vi "Launch Actors.vi"() -> ()   [LabVIEW 2020]
uses:
  Form Server.lvclass
  C:/Program Files (x86)/National Instruments/LabVIEW 2020/vi.lib/ActorFramework/Actor/Actor.lvclass
  Form Configuration.lvclass
  ADODB.lvclass
  C:/Users/User/Desktop/Raman Program/Database OOP/source/Database/Database.lvclass
  Working Range.lvclass
  Panel Form Controller.lvclass
  TRExperimentsRaw.lvclass
  DataSets.lvclass
  Sample Chemical Formula.lvclass
  Samples.lvclass
  Solutions.lvclass
  Users.lvclass
  Form Configuration.lvclass/Form Configuration.ctl
  Open Form Msg.lvclass/Open Form Msg.ctl
  <vilib>/ActorFramework/Message Enqueuer/Message Enqueuer.lvclass/Message Enqueuer.ctl
  <vilib>/ActorFramework/Message Enqueuer/Enqueue.vi
  <vilib>/MGI/Panel Manager/Panel/Panel/Window/Window.lvclass
  C:/Program Files (x86)/National Instruments/LabVIEW 2020/vi.lib/MGI/Panel Manager/Panel/Panel/Panel.lvclass
  Open Form Msg.lvclass
  C:/Program Files (x86)/National Instruments/LabVIEW 2020/vi.lib/ActorFramework/Message/Message.lvclass
  <vilib>/ActorFramework/Stop Msg/Stop Msg.lvclass
  <vilib>/MGI/Panel Manager/Panel/Panel/Window/Window.vi
  <vilib>/ActorFramework/Message Priority Queue/Priority Enqueue.vi
  <vilib>/ActorFramework/Actor/Actor.lvclass
  <vilib>/MGI/Panel Manager/Panel/Panel.lvlib
panel:
  in  "stop":bool
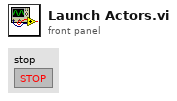
[diagram p1: front panel]
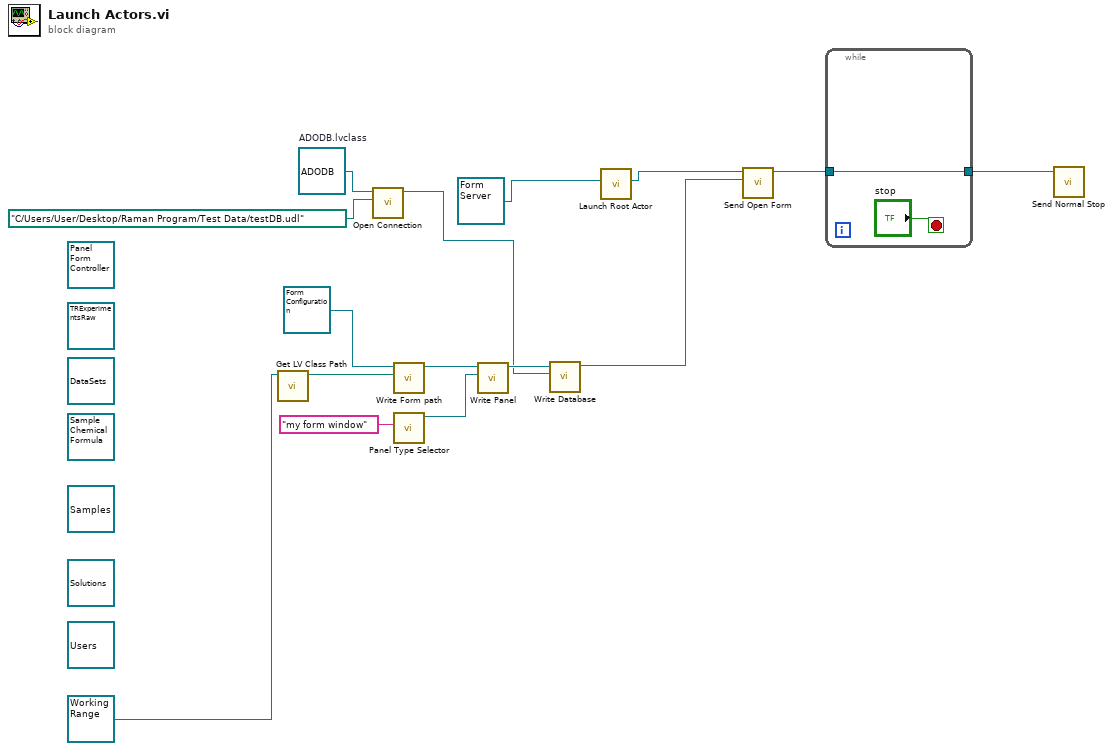
[diagram p0: block diagram]
diagram:
  (unwired) refnum<class "Users.lvclass"> refnum ("Forms.lvlib:Users.lvclass")
  (unwired) refnum<class "Solutions.lvclass"> refnum ("Forms.lvlib:Solutions.lvclass")
  (unwired) refnum<class "Samples.lvclass"> refnum ("Forms.lvlib:Samples.lvclass")
  (unwired) refnum<class "Sample Chemical Formula.lvclass"> refnum ("Forms.lvlib:Sample Chemical Formula.lvclass")
  (unwired) refnum<class "DataSets.lvclass"> refnum ("Forms.lvlib:DataSets.lvclass")
  w8 = refnum<class "ADODB.lvclass"> refnum  # ADODB.lvclass
  (unwired) refnum<class "TRExperimentsRaw.lvclass"> refnum ("Forms.lvlib:TRExperimentsRaw.lvclass")
  (unwired) refnum<class "Panel Form Controller.lvclass"> refnum ("Panel Form Controller.lvlib:Panel Form Controller.lvclass")
  n1 = call <vilib>:"Get LV Class Path.vi"("object"=refnum<class "Working Range.lvclass"> refnum ("Forms.lvlib:Working Range.lvclass")) -> ("class path"=w12:path)  [unwired: 9 in, 1 out]
  n2 = call-dynamic "Open Connection.vi"("Connection Info (Member Data/Prompt)"=path "C:/Users/User/Desktop/Raman Program/Test Data/testDB.udl", "ODBC in"=w8) -> ("ODBC out"=w1:refnum<class "ADODB.lvclass">)  [unwired: 8 in, 1 out]
  n3 = call "Write Form path.vi"("Form path"=w12, "Form Configuration in"=refnum<class "Form Configuration.lvclass"> refnum) -> ("Form Configuration out"=w13:refnum<class "Form Configuration.lvclass">)  [unwired: 8 in, 1 out]
  n4 = call-poly <vilib>:"Panel Type Selector.vi"("Default Title"="my form window") -> ("Window out"=w11:refnum<class "Window.lvclass">)  [unwired: 9 in, 1 out]
  n5 = call "Write Panel.vi"("Panel.lvlib:Panel.lvclass"=w11, "Form Configuration in"=w13) -> ("Form Configuration out"=w3:refnum<class "Form Configuration.lvclass">)  [unwired: 8 in, 1 out]
  n6 = call "Write Database.vi"("Database.lvclass"=w1, "Form Configuration in"=w3) -> ("Form Configuration out"=w2:refnum<class "Form Configuration.lvclass">)  [unwired: 8 in, 1 out]
  n7 = call <vilib>:"Launch Root Actor.vi"("Actor"=refnum<class "Form Server.lvclass"> refnum ("Form Server.lvlib:Form Server.lvclass")) -> ("Actor's Enqueuer"=w5:refnum<class "Message Enqueuer.lvclass">)  [unwired: 9 in, 1 out]
  n8 = call "Send Open Form.vi"("Form Config"=w2, "Message Enqueuer"=w5) -> ("Message Enqueuer out"=w4:refnum<class "Message Enqueuer.lvclass">)  [unwired: 8 in, 1 out]
  n9 = while {
    tunnel: w4 -> [w17]
    tunnel: [w17] -> w9
    stop <- "stop" stop-if-true
  }
  n10 = call <vilib>:"Send Normal Stop.vi"("Message Enqueuer"=w9) -> ()  [unwired: 10 in, 1 out]
